vi "Close Engine Reference.vi"(8 "error in (no error)":errorcluster, 11 "TestStand Engine":refnum<k7>) -> (0 "error out":errorcluster)   [LabVIEW 2010, in "TS Simple LabVIEW OI Dependencies.lvlib"]
uses:
  TS Simple LabVIEW OI Dependencies.lvlib
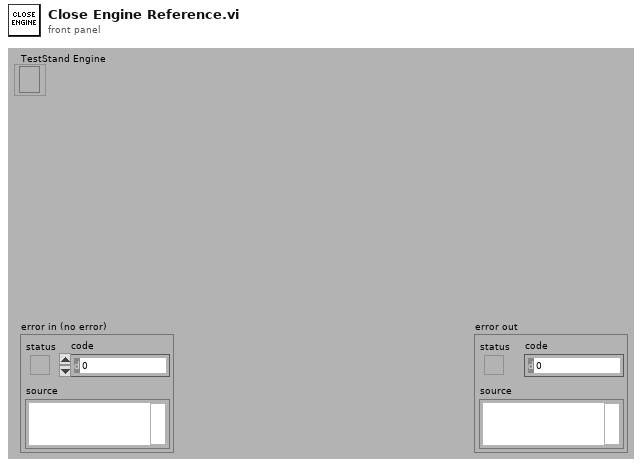
[diagram p1: front panel]
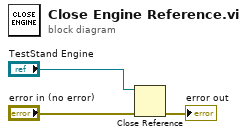
[diagram p0: block diagram]
diagram:
  n1 = Close Reference(reference="TestStand Engine", error in (no error)="error in (no error)") -> (error out=→"error out":errorcluster)
